vi "CreateSessionRequest.vi"(8 "error in (no error)":errorcluster, 11 "ModuleID":i32) -> (0 "error out":errorcluster)   [LabVIEW 2018, in "SensorModule.lvlib"]
uses:
  SensorModule.lvlib
  SensorShared/clEventType.ctl
  <vilib>/Utility/error.llb/Error Cluster From Error Code.vi
  <vilib>/ErrorRing/Error Ring.xnode
  SensorShared/SensorShared.lvlib
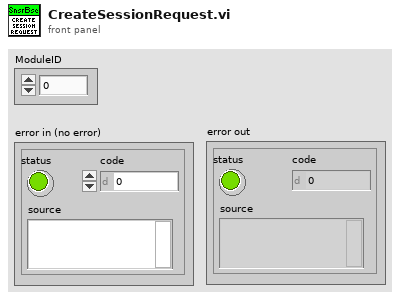
[diagram p1: front panel]
types:
  T1 = typedef "SensorShared.lvlib/clEventType.ctl" = cluster{"ModuleID":i32, "Data":variant}
  T2 = typedef "SensorShared.lvlib/clRequestEvents.ctl" = cluster{"StopRequest":refnum<user-event>, "PathToINI":refnum<user-event>, " LoadPlugin":refnum<user-event>, "ShowPanel":refnum<user-event>, "StartData":refnum<user-event>, "StopData":refnum<user-event>, "WriteConfig":refnum<user-event>, "ReadConfig":refnum<user-event>, "WriteEvtSignal":refnum<user-event>, "Configure":refnum<user-event>, "CreateSession":refnum<user-event>, "CloseSession":refnum<user-event>}
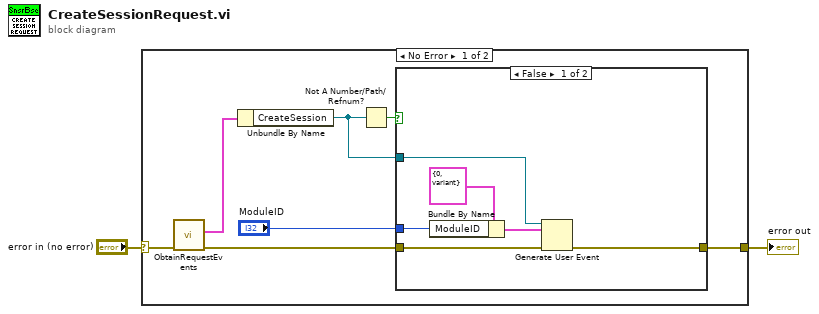
[diagram p0: block diagram]
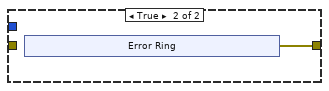
[diagram p2: hidden frame]
diagram:
  n1 = case shown="No Error" "error in (no error)" {
    selector: "error in (no error)" -> [w4 w22]
    tunnel: [w5 w22] -> w2
    frame No Error {
      n2 = call "ObtainRequestEvents.vi"("error in (no error)"=w4) -> ("error out"=w3:errorcluster, "clRequestEvents"=w9:T2)  [unwired: 9 in]
      n3 = Unbundle By Name(w9) -> ("CreateSession"=w7:refnum<user-event>)
      n4 = Not A Number/Path/Refnum?(number/path/refnum=w7) -> (NaN/Path/Refnum?=w8:bool)
      n5 = case shown="False" w8 {
        tunnel: w7 -> [w12 _]
        tunnel: "ModuleID" -> [w14 _]
        tunnel: [w11 w16] -> w5
        tunnel: w3 -> [w10 _]
        frame False {
          n6 = Bundle By Name(cluster=T1 {"ModuleID"=0, "Data"=variant} ("clEventType"), "ModuleID"=w14) -> (w13:T1)
          n7 = Generate User Event(user event=w12, event data cluster=w13, error in=w10) -> (error out=w11:errorcluster)  [unwired: 1 in, 1 out]
        }
        frame True {
          n8 = xnode "Error Ring"() -> ("error out"=w16:errorcluster)
        }
      }
    }
    frame Error {
    }
  }
  "error out" <- w2
